vi "Untitled 1 — копия.vi"() -> ()   [LabVIEW 2018]
uses:
  <vilib>/Utility/miscctls.llb/LVPoint32TypeDef.ctl
  <vilib>/Utility/miscctls.llb/LVPositionTypeDef.ctl
panel:
  out "reference out":refnum<vi>
  out "Position":T1
  out "Coords":T2
  in  "stop":bool
  out "Boolean 3":bool
  out "Boolean 2":bool
  out "Boolean":bool
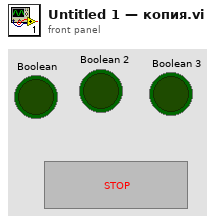
[diagram p1: front panel]
types:
  T1 = typedef "LVPositionTypeDef.ctl" = cluster{"Left":i32, "Top":i32}
  T2 = typedef "LVPoint32TypeDef.ctl" = cluster{"Horizontal":i32, "Vertical":i32}
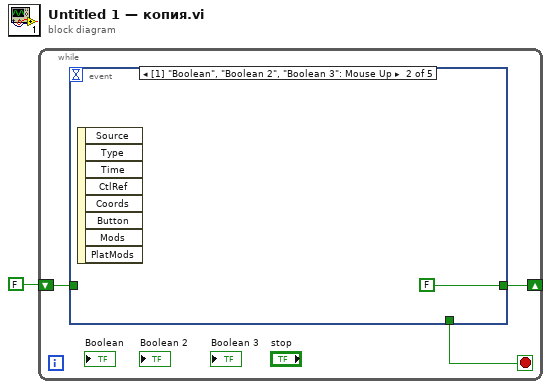
[diagram p0: block diagram]
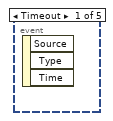
[diagram p2: hidden frame]
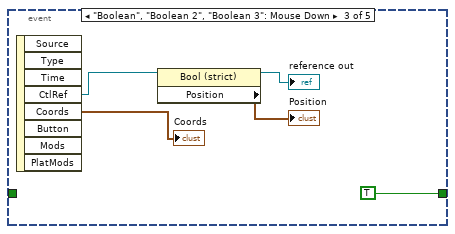
[diagram p3: hidden frame]
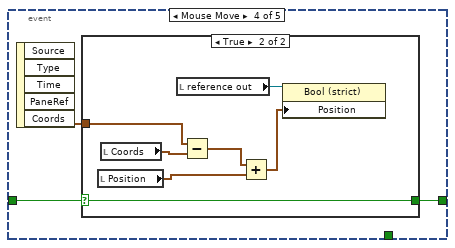
[diagram p4: hidden frame]
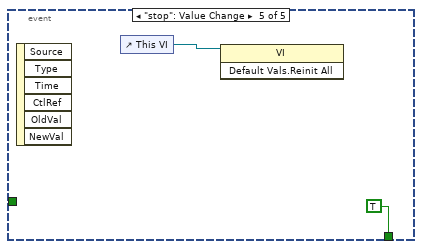
[diagram p6: hidden frame]
diagram:
  n1 = while {
    shift-right: [w3] -> _
    shift-left: FALSE -> [w4]
    stop <- w2 stop-if-true
    n2 = event shown="[1] \"Boolean\", \"Boolean 2\", \"Boolean 3\": Mouse Up" {
      selector: _ -> [_ _ _ _ _]
      dyn-events: _ -> [_ _ _ _ _]
      timeout: _ -> [_ _ _ _ _]
      tunnel: w4 -> [_ _ _ w12 _]
      tunnel: [_ FALSE TRUE w11 _] -> w3
      tunnel: [_ _ _ _ TRUE] -> w2
      event Timeout {
        n3 = event-data() -> ()  [unwired: 1 in, 3 out]
      }
      event "Boolean", "Boolean 2", "Boolean 3": Mouse Up {
        n4 = event-data() -> ()  [unwired: 1 in, 8 out]
      }
      event "Boolean", "Boolean 2", "Boolean 3": Mouse Down {
        n5 = event-data() -> ("CtlRef"=w10:refnum<vi>, "Coords"=→"Coords":T2)  [unwired: 1 in, 6 out]
        n6 = property class="Bool (strict)"(reference=w10) -> (reference out=→"reference out":refnum<vi>, "Position"=→"Position":T1)  [unwired: 1 in, 1 out]
      }
      event Mouse Move {
        n7 = event-data() -> ("Coords"=w13:T2)  [unwired: 1 in, 4 out]
        n8 = case shown="True" w12 {
          selector: w12 -> [w14 w15]
          tunnel: w13 -> [_ w21]
          tunnel: [w14 w15] -> w11
          frame False {
          }
          frame True {
            n9 = local read "Position"() -> (w18:T1)
            n10 = local read "Coords"() -> (w20:T2)
            n11 = local read "reference out"() -> (w17:refnum<vi>)
            n12 = Subtract(x=w21, y=w20) -> (x-y=w19:T2)
            n13 = Add(x=w19, y=w18) -> (x+y=w16:T2)
            n14 = property class="Bool (strict)"(reference=w17, "Position"=w16) -> ()  [unwired: 1 in, 2 out]
          }
        }
      }
      event "stop": Value Change {
        n15 = event-data() -> ()  [unwired: 1 in, 6 out]
        n16 = control-ref of="This VI"() -> (w22:refnum<vi>)
        n17 = invoke class="VI" method="Default Vals.Reinit All"(reference=w22) -> ()  [unwired: 2 in, 3 out]
      }
    }
  }
